vi "sv_Convert Value to String (Specific Datatype).vi"(7 "specific data type value":T1 items=["unknown"=0, "general"=1, "stress"=2, "strain"=3, "temperature"=5, "heat flux"=6, "displacement"=8, "reaction force"=9, "velocity"=11, "acceleration"=12, "excitation force"=13, "pressure"=15, "mass"=16, "time"=17, "frequency"=18, "rpm"=19, "order"=20, "sound pressure"=21, "sound intensity"=22, "sound power"=23]) -> (8 "specific data type string":string)   [LabVIEW 2017, in "SoundVib_UFF58.lvlib"]
uses:
  <vilib>/addons/Sound and Vibration/svt_UFF58/SoundVib_UFF58.lvlib
  <vilib>/addons/Sound and Vibration/svt_UFF58/subVIs/sv_UFF58 Specific Datatype.ctl
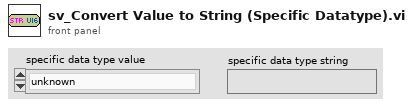
[diagram p1: front panel]
types:
  T1 = typedef "SoundVib_UFF58.lvlib/sv_UFF58 Specific Datatype.ctl" = u16
  T2 = typedef "SoundVib_UFF58.lvlib/sv_UFF58 Specific Datatype Array.ctl" = string[]
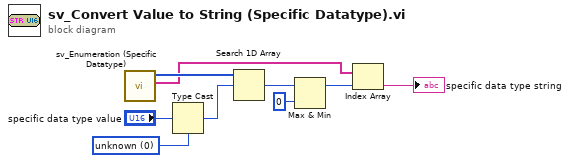
[diagram p0: block diagram]
diagram:
  w5 = u16 0 items=["unknown"=0, "general"=1, "stress"=2, "strain"=3, "temperature"=5, "heat flux"=6, "displacement"=8, "reaction force"=9, "velocity"=11, "acceleration"=12, "excitation force"=13, "pressure"=15, "mass"=16, "time"=17, "frequency"=18, "rpm"=19, "order"=20, "sound pressure"=21, "sound intensity"=22, "sound power"=23] ("specific data type string")
  n1 = call <vilib>:"sv_Enumeration (Specific Datatype).vi"() -> ("specific datatype strings"=w4:T2, "specific datatype U16 values"=w8:u16[])  [unwired: 10 in]
  n2 = Type Cast(type=w5, x="specific data type value") -> (*(type *) &x=w6:u16)
  n3 = Search 1D Array(1D array=w8, element=w6) -> (index of element=w3:i32)  [unwired: 1 in]
  n4 = Max & Min(x=w3, y=0) -> (max(x,y)=w2:i32)  [unwired: 1 out]
  n5 = Index Array(array=w4, index=w2) -> (element=→"specific data type string":string)
